vi "电池组信息组合.vi"(1 "数组":dbl[](array[numeric])) -> (0 "电池信息组合":dbl[](array[numeric]))   [LabVIEW 2013]
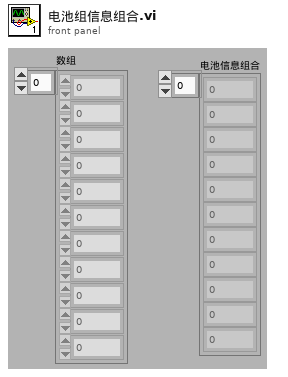
[diagram p1: front panel]
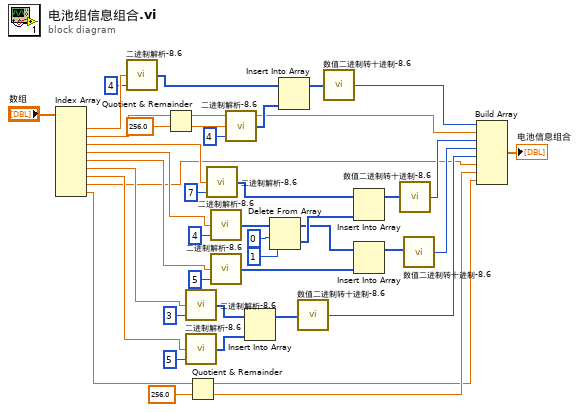
[diagram p0: block diagram]
diagram:
  n1 = Index Array(array="数组") -> (element #1=w42:dbl, element #2=w40:dbl, element #3=w30:dbl, element #4=w27:dbl, element #5=w26:dbl, element #6=w10:dbl, element #7=w9:dbl, element #8=w4:dbl, element #9=w13:dbl)  [unwired: 9 in]
  n2 = call "二进制解析-8.6.vi"("索引"=4, "数值"=w42) -> ("低位子数组"=w36:i32[])  [unwired: 3 out]
  n3 = Quotient & Remainder(x=w40, y=256.0) -> (x-y*floor(x/y)=w32:dbl, floor(x/y)=w37:dbl)
  n4 = call "二进制解析-8.6.vi"("索引"=3, "数值"=w10) -> ("低位子数组"=w8:i32[])  [unwired: 3 out]
  n5 = call "二进制解析-8.6.vi"("索引"=5, "数值"=w9) -> ("低位子数组"=w7:i32[])  [unwired: 3 out]
  n6 = Quotient & Remainder(x=w13, y=256.0) -> (x-y*floor(x/y)=w2:dbl, floor(x/y)=w3:dbl)
  n7 = call "二进制解析-8.6.vi"("索引"=7, "数值"=w30) -> ("低位子数组"=w22:i32[])  [unwired: 3 out]
  n8 = call "二进制解析-8.6.vi"("索引"=4, "数值"=w27) -> ("低位子数组"=w25:i32[])  [unwired: 3 out]
  n9 = call "二进制解析-8.6.vi"("索引"=5, "数值"=w26) -> ("低位子数组"=w19:i32[])  [unwired: 3 out]
  n10 = call "二进制解析-8.6.vi"("索引"=4, "数值"=w37) -> ("低位子数组"=w35:i32[])  [unwired: 3 out]
  n11 = Insert Into Array(array=w8, new element=w7) -> (w6:i32[])  [unwired: 1 in]
  n12 = Delete From Array(array=w25, length=0 ("索引"), index=1 ("长度")) -> (deleted portion=w21:i32[], array with subset deleted=w20:i32[])
  n13 = Insert Into Array(array=w36, new element=w35) -> (w34:i32[])  [unwired: 1 in]
  n14 = call "数值二进制转十进制-8.6.vi"("子数组"=w6) -> ("十进制数值"=w5:i32)  [unwired: 4 out]
  n15 = call "数值二进制转十进制-8.6.vi"("子数组"=w34) -> ("十进制数值"=w33:i32)  [unwired: 4 out]
  n16 = Insert Into Array(array=w22, new element=w21) -> (w17:i32[])  [unwired: 1 in]
  n17 = Insert Into Array(array=w20, new element=w19) -> (w18:i32[])  [unwired: 1 in]
  n18 = call "数值二进制转十进制-8.6.vi"("子数组"=w17) -> ("十进制数值"=w16:i32)  [unwired: 4 out]
  n19 = call "数值二进制转十进制-8.6.vi"("子数组"=w18) -> ("十进制数值"=w15:i32)  [unwired: 4 out]
  n20 = Build Array(w33, w32, w16, w15, w5, w4, w3, w2) -> (→"电池信息组合":dbl[])
